vi "Deserialize Picture Control Data.vi"(8 "error in (no error)":errorcluster, 11 "Layers in":refnum<class "Layer.lvclass">[](array[class])) -> (0 "error out":errorcluster, 3 "Layers out":refnum<class "Layer.lvclass">[](array[class]))   [LabVIEW 2021, in "lv_icon.lvlib"]
doc: "Every concentenate picture adds more and more data to the picture, therefore\nhis process is used to keep the picture memory amount as low as possible."
uses:
  <vilib>/LabVIEW Icon API/lv_icon/lv_icon.lvlib
  <vilib>/LabVIEW Icon API/lv_icon/Classes/Layer/Layer.lvclass
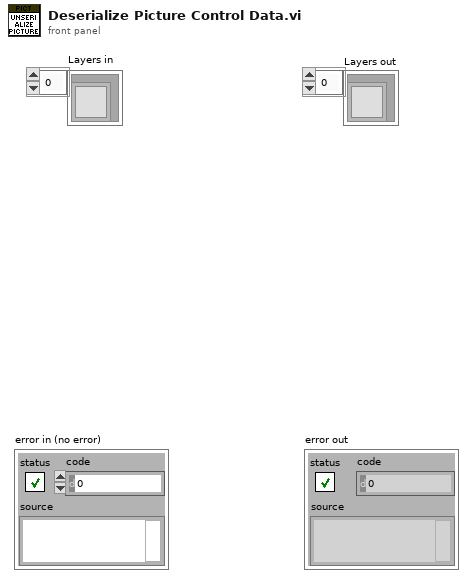
[diagram p1: front panel]
types:
  T1 = typedef "Layer.ctl" = cluster{"LayerIcon":picture, "LayerName":string, "Opacity":u8, "Visibility?":bool}
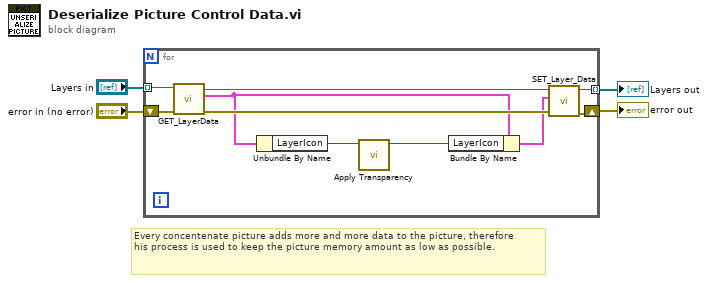
[diagram p0: block diagram]
diagram:
  # "Every concentenate picture adds more and more data to the picture, therefore\nhis process is used to keep the picture memory amount as low as possible."
  n1 = for {
    tunnel: "Layers in" -> [w14] mode=indexing
    tunnel: [w12] -> w3 mode=indexing
    shift-right: [w9] -> w1
    shift-left: "error in (no error)" -> [w11]
    n2 = call-dynamic "GET_LayerData.vi"("error in (no error)"=w11, "Layer.lvclass in"=w14) -> ("error out"=w10:errorcluster, "Data"=w8:T1, "Layer.lvclass out"=w13:refnum<class "Layer.lvclass">)  [unwired: 7 out]
    n3 = Unbundle By Name(w8) -> ("LayerIcon"=w6:picture)
    n4 = call <vilib>:"Apply Transparency.vi"("in"=w6) -> ("out"=w5:picture)  [unwired: 1 in, 9 out]
    n5 = Bundle By Name(cluster=w8, "LayerIcon"=w5) -> (w7:T1)
    n6 = call-dynamic "SET_Layer_Data.vi"("error in (no error)"=w10, "Data"=w7, "Layer.lvclass in"=w13) -> ("error out"=w9:errorcluster, "Layer.lvclass out"=w12:refnum<class "Layer.lvclass">)  [unwired: 1 in, 6 out]
  }
  "Layers out" <- w3
  "error out" <- w1
